vi "CleanWebCharacters.vi"(1 "string in":string) -> (0 "string out":string)   [LabVIEW 2024]
uses:
  <vilib>/Utility/error.llb/Trim Whitespace One-Sided.vi
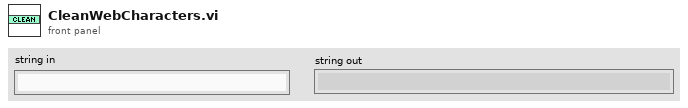
[diagram p1: front panel]
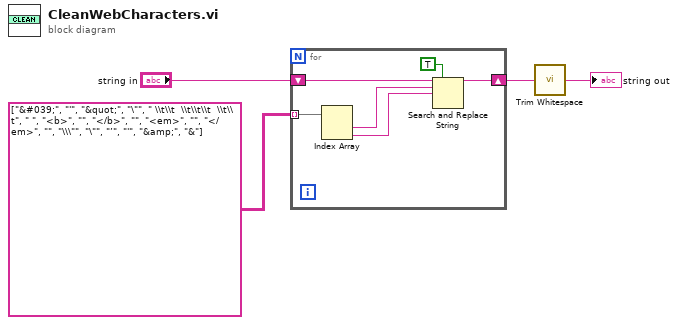
[diagram p0: block diagram]
diagram:
  n1 = for {
    tunnel: string[][] [["&#039;", "'"], ["&quot;", "\""], [" \\t\\t  \\t\\t\\t  \\t\\t", " "], ["<b>", ""], ["</b>", ""], ["<em>", ""], ["</em>", ""], ["\\\"", "\""], ["’", "'"], ["&amp;", "&"]] -> [w10] mode=indexing
    shift-right: [w8] -> w2
    shift-left: "string in" -> [w9]
    n2 = Index Array(array=w10) -> (element #1=w6:string, element #2=w5:string)  [unwired: 2 in]
    n3 = Search and Replace String(replace all?=TRUE ("replace all? (F)"), input string=w9, search string=w6, replace string=w5) -> (result string=w8:string)  [unwired: 4 in, 3 out]
  }
  n4 = call <vilib>:"Trim Whitespace.vi"("string"=w2) -> ("trimmed string"=→"string out":string)  [unwired: 1 in]
